vi "Read Pages.vi"(8 "Error In":errorcluster caption="error in", 11 "Custom Device Page .NET Ref In":refnum<k24>) -> (0 "Error Out":errorcluster caption="error in", 2 "All Pages Properties":T8(array[cluster]), 3 "Custom Device Page .NET Ref Out":refnum<k24>)   [LabVIEW 2019, in "VeriStand Custom Device XML Parser.lvlib"]
doc: "Reads and returns the properties for all pages of the custom device"
uses:
  VeriStand Custom Device XML Parser.lvlib
  NationalInstruments.VeriStand.XMLReader
  XML Controls/Path Cluster.ctl
  XML Controls/Help File Properties.ctl
  XML Controls/Button Properties.ctl
  XML Controls/Button Type.ctl
  XML Controls/Dependency Properties.ctl
  XML Controls/RuntTimeMenu Properties.ctl
  XML Controls/Execution Types.ctl
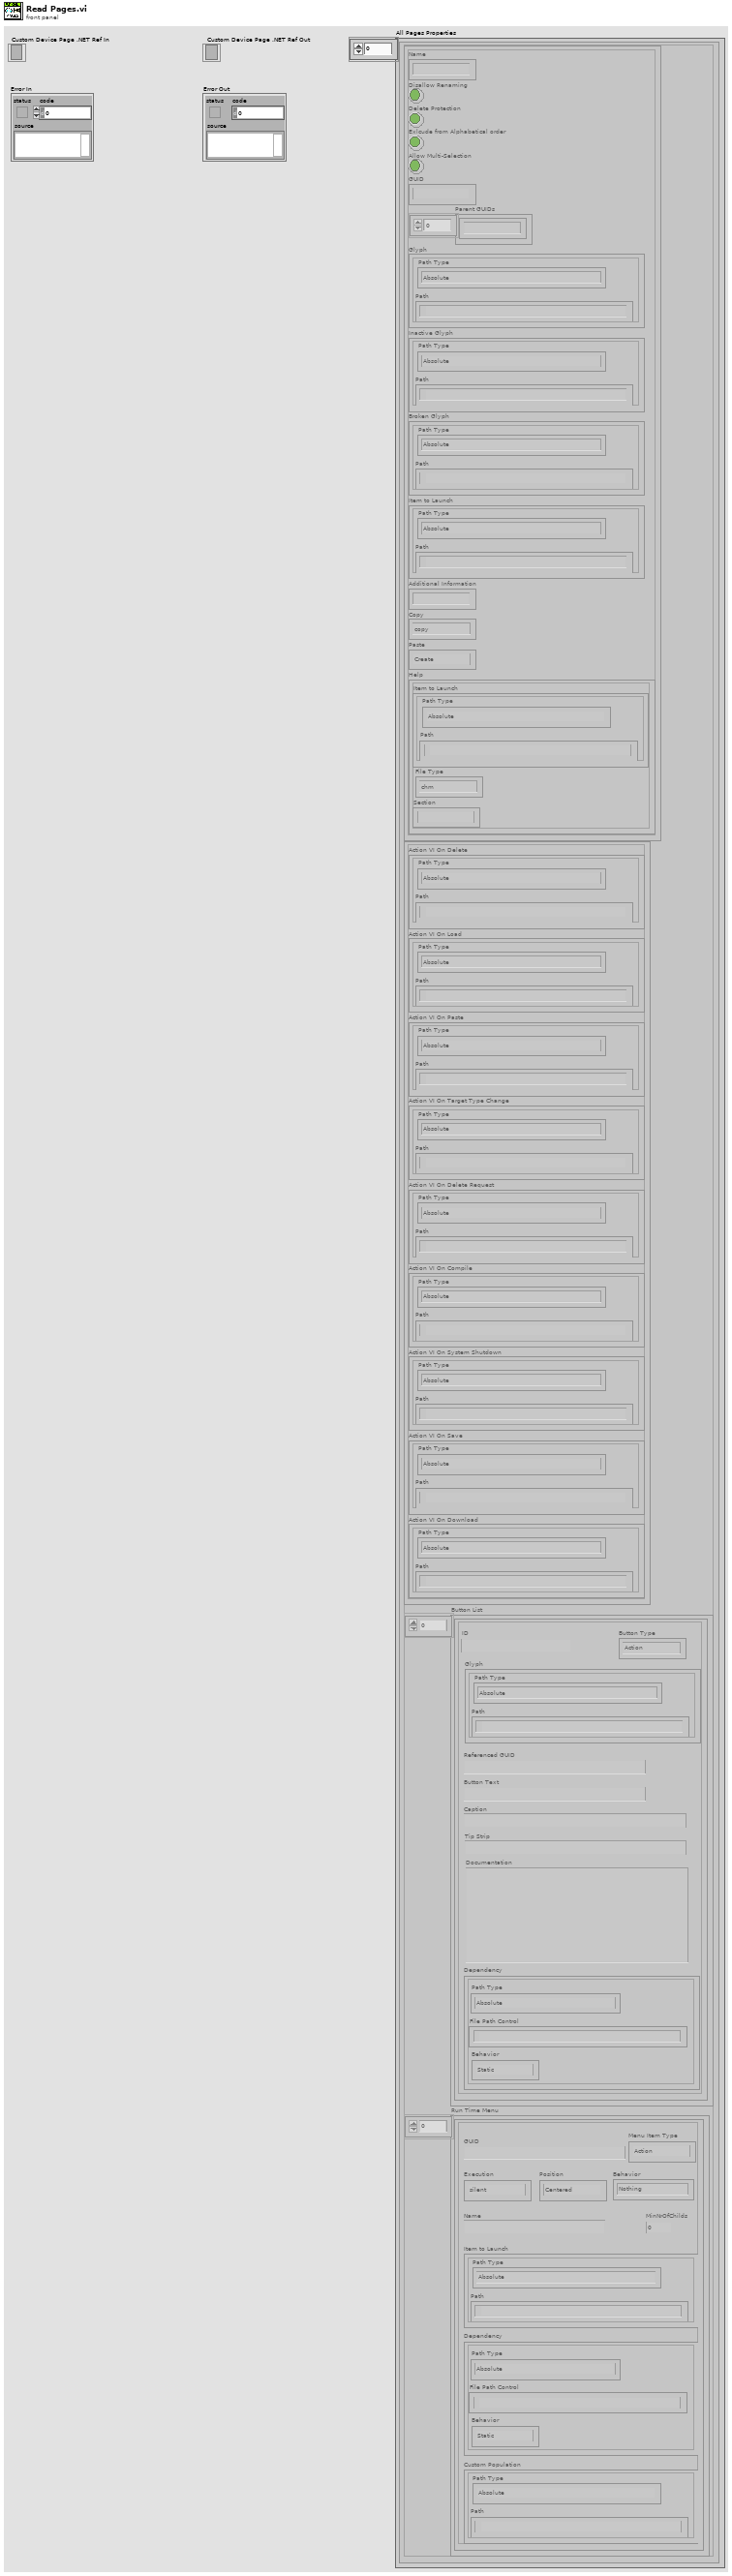
[diagram p1: front panel]
types:
  T1 = typedef "VeriStand Custom Device XML Parser.lvlib/Path Cluster.ctl" = cluster{"Path":path, "Path Type":enum16{"Absolute", "To Base", "To Common Doc Dir", "To Application Data Dir"}}
  T2 = typedef "VeriStand Custom Device XML Parser.lvlib/Help File Properties.ctl" = cluster{"Item to Launch":T1, "Section":string, "File Type":enum16{"chm", "other"}}
  T3 = typedef "VeriStand Custom Device XML Parser.lvlib/Button Properties.ctl" = cluster{"ID":string, "Glyph":T1, "Button Type":T4, "Referenced GUID":string, "Button Text":string, "Caption":string, "Tip Strip":string, "Documentation":string, "Dependency":T5}
  T4 = typedef "VeriStand Custom Device XML Parser.lvlib/Button Type.ctl" = enum16{"Action", "Dialog", "Page", "Notification", "Separator"}
  T5 = typedef "VeriStand Custom Device XML Parser.lvlib/Dependency Properties.ctl" = cluster{"File Path Control":path, "Path Type":enum16{"Absolute", "To Base", "To Common Doc Dir", "To Application Data Dir"}, "Behavior":enum16{"Static", "Dynamic"}}
  T6 = typedef "VeriStand Custom Device XML Parser.lvlib/RuntTimeMenu Properties.ctl" = cluster{"GUID":string, "Execution":T7, "MinNrOfChilds":u32, "Name":string, "Item to Launch":T1, "Dependency":T5, "Custom Population":T1, "Menu Item Type":enum16{"Action", "VI", "Separator", "Custom"}, "Behavior":enum16{"Nothing", "Open Front Panel"}, "Position":enum16{"Centered", "Mouse Pointer"}}
  T7 = typedef "VeriStand Custom Device XML Parser.lvlib/Execution Types.ctl" = enum16{"silent", "modal", "floating", "default"}
  T8 = cluster{"Cluster":cluster{"Name":string, "Disallow Renaming":bool, "Delete Protection":bool, "Exlcude from Alphabetical order":bool, "Allow Multi-Selection":bool, "GUID":string, "Parent GUIDs":string[], "Glyph":T1, "Inactive Glyph":T1, "Broken Glyph":T1, "Item to Launch":T1, "Additional Information":string, "Copy":enum16{"copy", "disabled"}, "Paste":enum16{"Create", "CreatIfNotExists_GUID", "CreatIfNotExists_Name", "Replace", "Dialog"}, "Help":T2}, "Cluster":cluster{"Action VI On Delete":T1, "Action VI On Load":T1, "Action VI On Paste":T1, "Action VI On Target Type Change":T1, "Action VI On Delete Request":T1, "Action VI On Compile":T1, "Action VI On System Shutdown":T1, "Action VI On Save":T1, "Action VI On Download":T1}, "Button List":T3[], "Run Time Menu":T6[]}[]
  T9 = cluster{"General Properties":cluster{"Name":string, "Disallow Renaming":bool, "Delete Protection":bool, "Exlcude from Alphabetical order":bool, "Allow Multi-Selection":bool, "GUID":string, "Parent GUIDs":string[], "Glyph":T1, "Inactive Glyph":T1, "Broken Glyph":T1, "Item to Launch":T1, "Additional Information":string, "Copy":enum16{"copy", "disabled"}, "Paste":enum16{"Create", "CreatIfNotExists_GUID", "CreatIfNotExists_Name", "Replace", "Dialog"}, "Help":T2}, "ActionVI Properties":cluster{"Action VI On Delete":T1, "Action VI On Load":T1, "Action VI On Paste":T1, "Action VI On Target Type Change":T1, "Action VI On Delete Request":T1, "Action VI On Compile":T1, "Action VI On System Shutdown":T1, "Action VI On Save":T1, "Action VI On Download":T1}, "Button List Properties":T3[], "Run Time Menu  Properties":T6[]}
  T10 = cluster{"Name":string, "Disallow Renaming":bool, "Delete Protection":bool, "Exlcude from Alphabetical order":bool, "Allow Multi-Selection":bool, "GUID":string, "Parent GUIDs":string[], "Glyph":T1, "Inactive Glyph":T1, "Broken Glyph":T1, "Item to Launch":T1, "Additional Information":string, "Copy":enum16{"copy", "disabled"}, "Paste":enum16{"Create", "CreatIfNotExists_GUID", "CreatIfNotExists_Name", "Replace", "Dialog"}, "Help":T2}
  T11 = cluster{"Action VI On Delete":T1, "Action VI On Load":T1, "Action VI On Paste":T1, "Action VI On Target Type Change":T1, "Action VI On Delete Request":T1, "Action VI On Compile":T1, "Action VI On System Shutdown":T1, "Action VI On Save":T1, "Action VI On Download":T1}
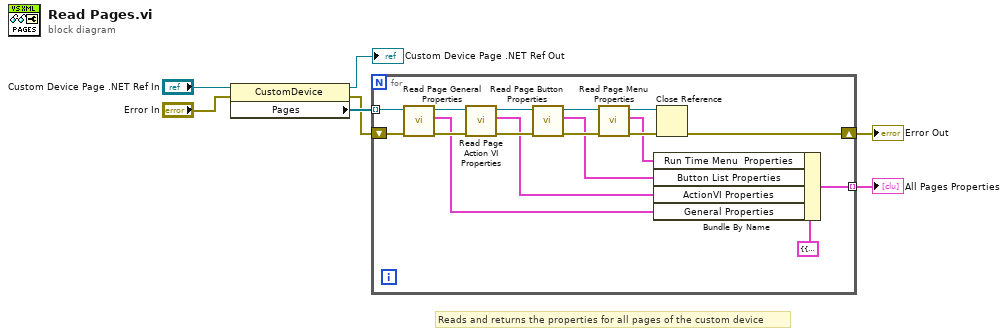
[diagram p0: block diagram]
diagram:
  # "Reads and returns the properties for all pages of the custom device"
  n1 = property class="CustomDevice"(reference="Custom Device Page .NET Ref In", error in="Error In") -> (reference out=→"Custom Device Page .NET Ref Out":refnum<k24>, error out=w3:errorcluster, "Pages"=w4:refnum<k24>[])
  n2 = for {
    tunnel: w4 -> [w24] mode=indexing
    shift-right: [w9] -> w1
    shift-left: w3 -> [w23]
    tunnel: [w8] -> w2 mode=indexing
    n3 = call "Read Page General Properties.vi"("Error In"=w23, "Custom Device Page .NET Ref In"=w24) -> ("Error Out"=w21:errorcluster, "General Page Properties"=w10:T10, "Custom Device Page .NET Ref Out"=w22:refnum<k24>)  [unwired: 7 in]
    n4 = call "Read Page Action VI Properties.vi"("Error In"=w21, "Custom Device Page .NET Ref In"=w22) -> ("Error Out"=w19:errorcluster, "ActionVI Properties"=w11:T11, "Custom Device Page .NET Ref Out"=w20:refnum<k24>)  [unwired: 7 in]
    n5 = call "Read Page Button Properties.vi"("Error In"=w19, "Custom Device Page .NET Ref In"=w20) -> ("Error Out"=w17:errorcluster, "All Button Properties"=w12:T3[], "Custom Device Page .NET Ref Out"=w18:refnum<k24>)  [unwired: 7 in]
    n6 = call "Read Page Menu Properties.vi"("Error In"=w17, "Custom Device Page .NET Ref In"=w18) -> ("Error Out"=w16:errorcluster, "All Menu Properties"=w13:T6[], "Custom Device Page .NET Ref Out"=w15:refnum<k24>)  [unwired: 7 in]
    n7 = Bundle By Name(cluster=T9 {"General Properties"={"Name"="", "Disallow Renaming"=FALSE, "Delete Protection"=FALSE, "Exlcude from Alphabetical order"=FALSE, "Allow Multi-Selection"=FALSE, "GUID"="", "Parent GUIDs"=[], "Glyph"={"Path"=path "", "Path Type"=enum."Absolute"}, "Inactive Glyph"={"Path"=path "", "Path Type"=enum."Absolute"}, "Broken Glyph"={"Path"=path "", "Path Type"=enum."Absolute"}, "Item to Launch"={"Path"=path "", "Path Type"=enum."Absolute"}, "Additional Information"="", "Copy"=enum."copy", "Paste"=enum."Create", "Help"={"Item to Launch"={"Path"=path "", "Path Type"=enum."Absolute"}, "Section"="", "File Type"=enum."chm"}}, "ActionVI Properties"={"Action VI On Delete"={"Path"=path "", "Path Type"=enum."Absolute"}, "Action VI On Load"={"Path"=path "", "Path Type"=enum."Absolute"}, "Action VI On Paste"={"Path"=path "", "Path Type"=enum."Absolute"}, "Action VI On Target Type Change"={"Path"=path "", "Path Type"=enum."Absolute"}, "Action VI On Delete Request"={"Path"=path "", "Path Type"=enum."Absolute"}, "Action VI On Compile"={"Path"=path "", "Path Type"=enum."Absolute"}, "Action VI On System Shutdown"={"Path"=path "", "Path Type"=enum."Absolute"}, "Action VI On Save"={"Path"=path "", "Path Type"=enum."Absolute"}, "Action VI On Download"={"Path"=path "", "Path Type"=enum."Absolute"}}, "Button List Properties"=[], "Run Time Menu  Properties"=[]} ("Cluster"), "Run Time Menu  Properties"=w13, "Button List Properties"=w12, "ActionVI Properties"=w11, "General Properties"=w10) -> (w8:T9)
    n8 = Close Reference(reference=w15, error in (no error)=w16) -> (error out=w9:errorcluster)
  }
  "Error Out" <- w1
  "All Pages Properties" <- w2
